vi "Launcher Builder.vi"   [LabVIEW 2021]
uses:
  SuperVolatus/Libs/lv-builder/Builder Tools/Builder/Builder.lvclass
  SuperVolatus/Libs/lv-builder/Builder Tools/Simple Build GUI/Simple Build GUI.lvclass
panel:
  # "LAUNCHER\nBuilder"
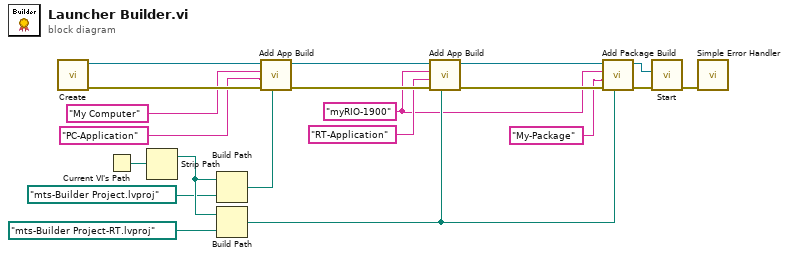
[diagram p0: block diagram]
diagram:
  w2 = "myRIO-1900" ("Target")
  n1 = call "Create.vi"() -> ("error out"=w14:errorcluster, "Builder out"=w15:refnum<class "Builder.lvclass">)  [unwired: 10 in]
  n2 = Current VI's Path() -> (path=w17:path)
  n3 = Strip Path(path=w17) -> (stripped path=w20:path)  [unwired: 1 out]
  n4 = Build Path(base path=w20, name or relative path=path "mts-Builder Project.lvproj") -> (appended path=w4:path)
  n5 = Build Path(base path=w20, name or relative path=path "mts-Builder Project-RT.lvproj") -> (appended path=w3:path)
  n6 = call "Add App Build.vi"("Project Path (Autodetect)"=w4, "error in (no error)"=w14, "Build Spec"="PC-Application" ("Target"), "Target"="My Computer", "Builder in"=w15) -> ("error out"=w12:errorcluster, "Builder out"=w13:refnum<class "Builder.lvclass">)  [unwired: 5 in]
  n7 = call "Add App Build.vi"("Project Path (Autodetect)"=w3, "error in (no error)"=w12, "Build Spec"="RT-Application" ("Target"), "Target"=w2, "Builder in"=w13) -> ("error out"=w10:errorcluster, "Builder out"=w11:refnum<class "Builder.lvclass">)  [unwired: 5 in]
  n8 = call "Add Package Build.vi"("Project Path (Autodetect)"=w3, "error in (no error)"=w10, "Build Spec"="My-Package" ("Target"), "Target"=w2, "Builder in"=w11) -> ("error out"=w9:errorcluster, "Builder out"=w1:refnum<class "Builder.lvclass">)  [unwired: 5 in]
  n9 = call "Start.vi"("error in (no error)"=w9, "Builder"=w1) -> ("error out"=w16:errorcluster)  [unwired: 8 in, 1 out]
  n10 = call <vilib>:"Simple Error Handler.vi"("error in (no error)"=w16) -> ()  [unwired: 4 in, 5 out]
